vi "Unknown Case.vi"(8 "error in (no error)":errorcluster, 10 "source":string, 11 "case":string) -> (0 "error out":errorcluster)   [LabVIEW 2020]
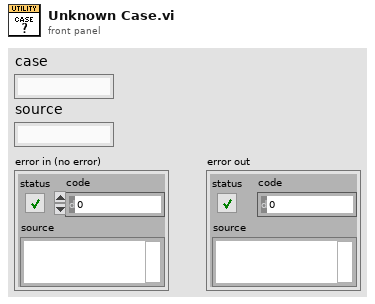
[diagram p1: front panel]
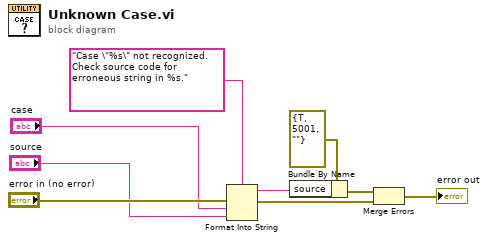
[diagram p0: block diagram]
diagram:
  n1 = Format Into String(format string="Case \"%s\" not recognized. Check source code for erroneous string in %s.", error in="error in (no error)", "case", "source") -> (resulting string=w6:string, error out=w3:errorcluster)  [unwired: 1 in]
  n2 = Bundle By Name(cluster=errorcluster {"status"=TRUE, "code"=5001, "source"=""} ("error out"), "source"=w6) -> (w1:errorcluster)
  n3 = Merge Errors(w1, w3) -> (→"error out":errorcluster)
